vi "导出曲线数组.vi"(0 "压力参数":dbl[](array[numeric]), 1 "位移参数":dbl[](array[numeric]), 5 "file path (dialog if empty)":path caption="文件路径 （空时为对话框）") -> ()   [LabVIEW 2013]
uses:
  <vilib>/Utility/file.llb/Write To Spreadsheet File (DBL).vi
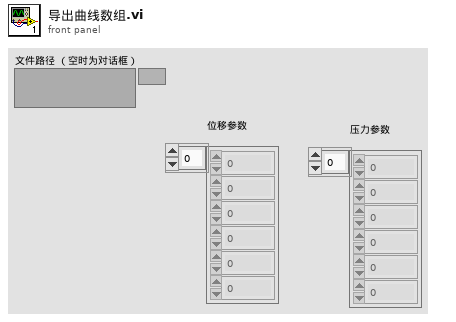
[diagram p1: front panel]
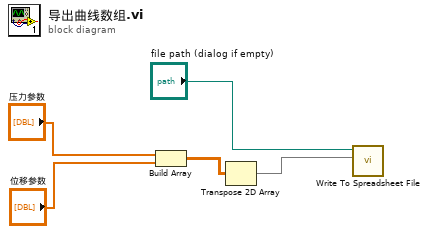
[diagram p0: block diagram]
diagram:
  n1 = Build Array("压力参数", "位移参数") -> (w5:dbl[][])
  n2 = Transpose 2D Array(2D array=w5) -> (transposed array=w4:dbl[][])
  n3 = call-poly <vilib>:"Write To Spreadsheet File.vi"("2D data"=w4, "file path (dialog if empty)"="file path (dialog if empty)") -> ()  [unwired: 6 in, 1 out]
